vi "ReceiveTimeStampData.vi"(6 "Timeout ms":i32=1, 7 "UDPTimestamp":T2) -> (0 "error out":errorcluster, 1 "TimeStampData":cluster{"time":string}, 2 "Did Receive":bool, 3 "UDP Output":T1)   [LabVIEW 2019]
panel:
  # "Receive Port"
  # "Send Port"
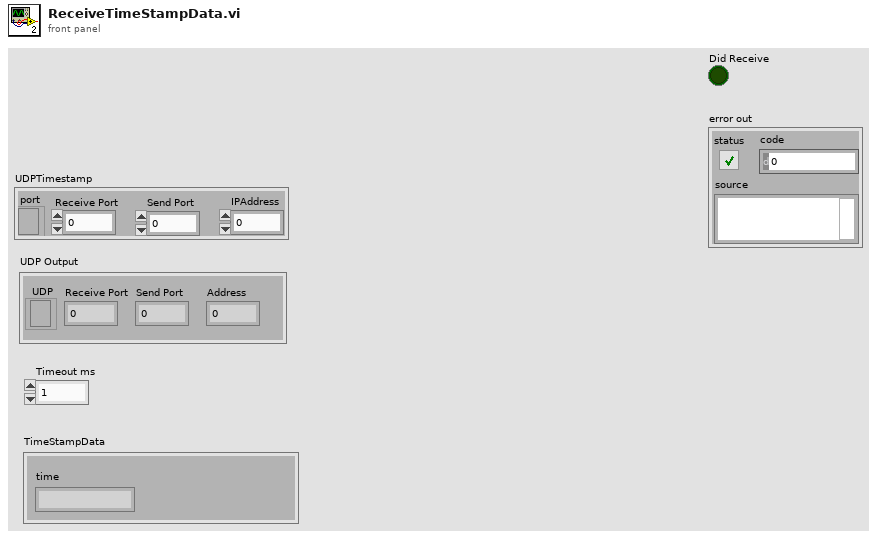
[diagram p1: front panel]
types:
  T1 = cluster{"UDP":refnum<k16>, "Receive Port":i32, "Send Port":i32, "Address":i64}
  T2 = cluster{"port":refnum<k16>, i32, i32, "IPAddress":i64}
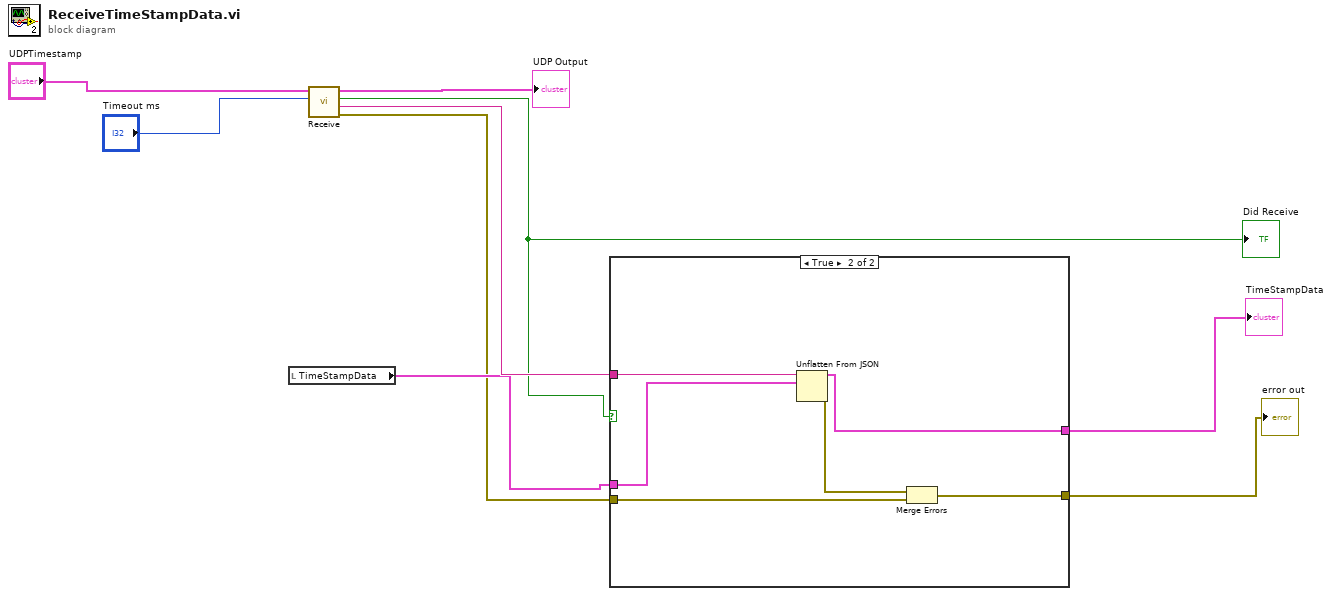
[diagram p0: block diagram]
diagram:
  n1 = local read "TimeStampData"() -> (w4:cluster{"time":string})
  n2 = call "Receive.vi"("Timeout ms"="Timeout ms", "UDP Input"="UDPTimestamp") -> ("Error Out"=w3:errorcluster, "Received Data"=w6:string, "Did Receive"=w1:bool, "UDP Output"=→"UDP Output":T1)  [unwired: 2 in]
  "Did Receive" <- w1
  n3 = case shown="True" w1 {
    tunnel: w6 -> [_ w17]
    tunnel: [w10 w16] -> w5
    tunnel: w4 -> [w10 w15]
    tunnel: w3 -> [w11 w14]
    tunnel: [w11 w13] -> w2
    frame False {
    }
    frame True {
      n4 = Unflatten From JSON(JSON string=w17, type and defaults=w15) -> (value=w16:cluster{"time":string}, error out=w12:errorcluster)  [unwired: 5 in]
      n5 = Merge Errors(w12, w14) -> (w13:errorcluster)
    }
  }
  "TimeStampData" <- w5
  "error out" <- w2
